vi "getWaypoints.vi"(8 "error in (no error)":errorcluster, 11 "GoTo in":refnum<class "GoTo.lvclass">) -> (0 "error out":errorcluster, 2 "Waypoint Array":refnum<class "Waypoint.lvclass">[](array[class]), 3 "GoTo out":refnum<class "GoTo.lvclass">)   [LabVIEW 2013, in "GoTo.lvclass"]
uses:
  GoTo.lvclass
  Waypoint/Waypoint.lvclass
  GoTo.lvclass/GoTo.ctl
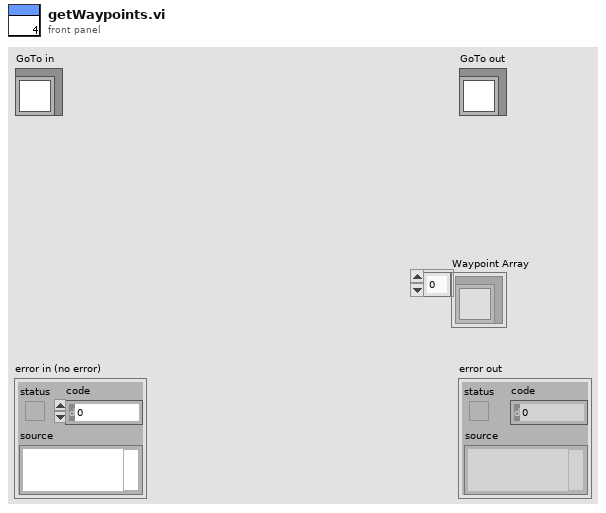
[diagram p1: front panel]
types:
  T1 = typedef "UTM Location.ctl" = cluster{"UTM Zone":dbl, "Hemisphere":enum16{"North", "South"}, "East":dbl, "North":dbl}
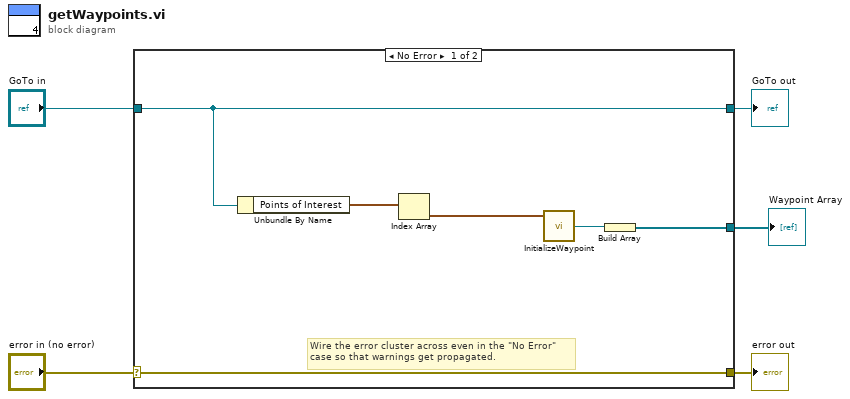
[diagram p0: block diagram]
diagram:
  n1 = case shown="No Error" "error in (no error)" {
    selector: "error in (no error)" -> [w11 w13]
    tunnel: [w11 w13] -> w4
    tunnel: [w10 w12] -> w2
    tunnel: "GoTo in" -> [w10 w12]
    tunnel: [w6 _] -> w1
    frame No Error {
      # "Wire the error cluster across even in the \"No Error\"\ncase so that warnings get propagated."
      n2 = Unbundle By Name(w10) -> ("Points of Interest"=w9:T1[])
      n3 = Index Array(array=w9) -> (element=w8:T1)  [unwired: 1 in]
      n4 = call "InitializeWaypoint.vi"("Coords"=w8) -> ("Waypoint Out"=w7:refnum<class "Waypoint.lvclass">)  [unwired: 2 in]
      n5 = Build Array(w7) -> (w6:refnum<class "Waypoint.lvclass">[])
    }
    frame Error {
    }
  }
  "error out" <- w4
  "GoTo out" <- w2
  "Waypoint Array" <- w1
